vi "SVGen (FXP).vi"(7 "PWM  (Period)":fxp<+,32,10>, 8 "1/Vdc":fxp<+/-,16,10> format="%.16g", 9 "Vr3":fxp<+/-,32,12>, 10 "Vr2":fxp<+/-,32,12>, 11 "Vr1":fxp<+/-,32,12>) -> (0 "Tc":fxp<+/-,37,17> format="%.26g", 1 "PWM3":fxp<+,16,16>, 2 "PWM2":fxp<+,16,16>, 3 "PWM1":fxp<+,16,16>, 4 "Tb":fxp<+/-,37,17> format="%.26g", 5 "number":u8, 6 "Ta":fxp<+/-,37,17> format="%.26g")   [LabVIEW 2025]
uses:
  <vilib>/rvi/FXPMathLib/FxpMul/XNode/nifxpmath_Multiplier.xnode
  <vilib>/rvi/FXPMathLib/sim/FxpSim.dll
  <vilib>/Platform/TimedLoop/XDataNode/wakeup.ctl
  <vilib>/Platform/TimedLoop/XDataNode/XDNodeRunTimeDep.lvlib
  <vilib>/Platform/TimedLoop/XDataNode/nitl_modes.ctl
  <vilib>/Platform/TimedLoop/XDataNode/timing_clust.ctl
  <vilib>/platform/TimedLoop/XDataNode/XDataNode.xnode
  <vilib>/rvi/FXPMathLib/FxpAdd/XNode/nifxpmath_Add.xnode
panel:
  out "number":u8
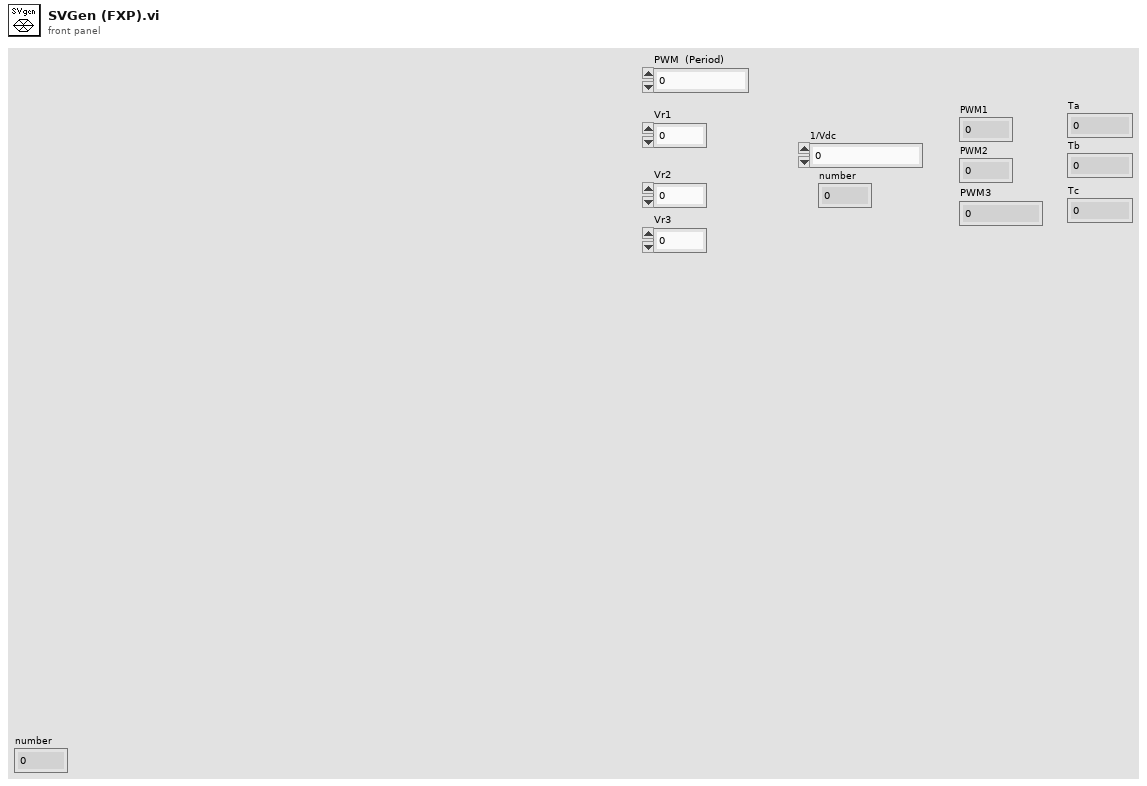
[diagram p1: front panel]
types:
  T1 = typedef "XDNodeRunTimeDep.lvlib/timing_clust.ctl" = cluster{"Expected End [f-1]":u64, "Actual End [f-1]":u64, "Finished Late? [f-1]":bool, "Expected End [i-1]":u64, "Actual End [i-1]":u64, "Finished Late? [i-1]":bool, "Expected Start [i]":u64, "Actual Start [i]":u64, "Expected Start [f]":u64, "Actual Start [f]":u64, "Source Name":string, "Structure Name":string, "Period":i64, "Deadline":i64, "Offset":i64, "Start":i64, "Priority":i32, "Timeout":i32, "Mode":T2, "Wakeup Reason":T3, "Error":errorcluster, "Source Type":string, "Secondary Source Type":string, "Global End Time":u64, "Global Start Time":u64, "Frame Duration":u64, "Iteration Duration":u64, "Assigned CPU":i32, "I/O Scan Engine Mode":u32}
  T2 = typedef "XDNodeRunTimeDep.lvlib/nitl_modes.ctl" = enum32{"No Change", "Process missed periods, maintain original phase", "Discard missed periods, maintain original phase", "Process missed periods, ignore original phase", "Discard missed periods, ignore original phase"}
  T3 = typedef "XDNodeRunTimeDep.lvlib/wakeup.ctl" = enum32{"Normal", "Aborted", "Asynchronous wakeup", "Timing source error", "Timed loop error", "Timeout"}
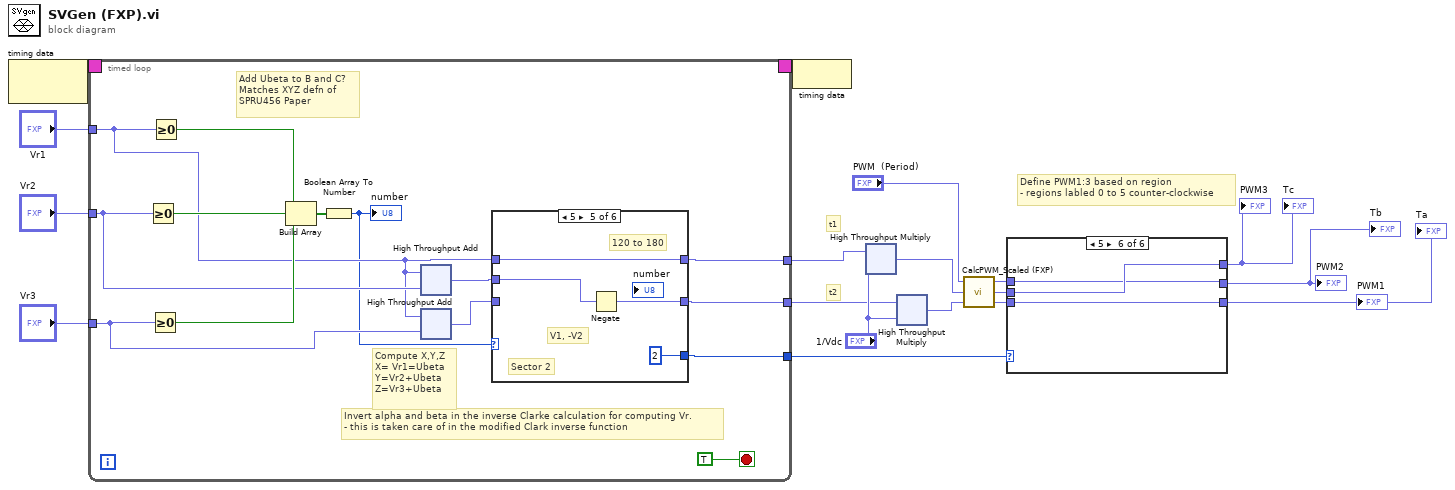
[diagram p0: block diagram]
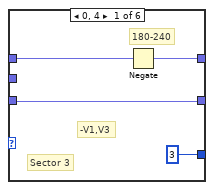
[diagram p2: hidden frame]
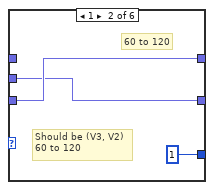
[diagram p3: hidden frame]
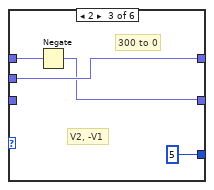
[diagram p4: hidden frame]
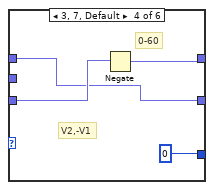
[diagram p5: hidden frame]
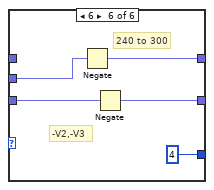
[diagram p6: hidden frame]
diagram:
  # "t2"
  # "t1"
  # "Define PWM1:3 based on region\n- regions labled 0 to 5 counter-clockwise"
  n1 = node-c288() -> (w18:T1)  [unwired: 1 out]
  n2 = timed-loop {
    timing: w18 -> [_]
    timing-out: [_] -> w17
    tunnel: [w20] -> w3
    tunnel: [w21] -> w7
    tunnel: [w22] -> w9
    tunnel: "Vr2" -> [w28]
    tunnel: "Vr1" -> [w25]
    tunnel: "Vr3" -> [w27]
    stop <- TRUE stop-if-true
    # "Compute X,Y,Z\nX= Vr1=Ubeta\nY=Vr2+Ubeta\nZ=Vr3+Ubeta"
    # "Add Ubeta to B and C?\nMatches XYZ defn of \nSPRU456 Paper"
    # "Invert alpha and beta in the inverse Clarke calculation for computing Vr.\n- this is taken care of in the modified Clark inverse function"
    n3 = Greater Or Equal To 0?(x=w28) -> (x >= 0?=w30:bool)
    n4 = Greater Or Equal To 0?(x=w27) -> (x >= 0?=w29:bool)
    n5 = Greater Or Equal To 0?(x=w25) -> (x >= 0?=w31:bool)
    n6 = Build Array(w31, w30, w29) -> (w32:bool[])
    n7 = Boolean Array To Number(Boolean array=w32) -> (number=w19:u8)
    "number" <- w19
    n8 = xnode "High Throughput Add"("x"=w25, "y"=w28) -> ("x+y"=w24:fxp<+/-,32,12>)
    n9 = xnode "High Throughput Add"("x"=w25, "y"=w27) -> ("x+y"=w23:fxp<+/-,32,12>)
    n10 = case shown="5" w19 {
      tunnel: [w36 w38 w41 w45 w50 w54] -> w22
      tunnel: w24 -> [_ w37 w41 _ w49 w55]
      tunnel: w23 -> [w33 w38 _ w46 _ w52]
      tunnel: [w33 w37 w40 w44 w48 w53] -> w21
      tunnel: w25 -> [w34 _ w42 w44 w50 _]
      tunnel: [3 1 5 0 2 4] -> w20
      frame 0, 4 {
        # "Sector 3"
        # "-V1,V3"
        # "180-240"
        n11 = Negate(x=w34) -> (-x=w36:fxp<+/-,33,13>)
      }
      frame 1 {
        # "Should be (V3, V2)\n60 to 120"
        # "60 to 120"
      }
      frame 2 {
        # "V2, -V1"
        # "300 to 0"
        n12 = Negate(x=w42) -> (-x=w40:fxp<+/-,33,13>)
      }
      frame 3, 7, Default {
        # "V2,-V1"
        # "0-60"
        n13 = Negate(x=w46) -> (-x=w45:fxp<+/-,33,13>)
      }
      frame 5 {
        # "Sector 2"
        # "V1, -V2"
        # "120 to 180"
        n14 = Negate(x=w49) -> (-x=w48:fxp<+/-,33,13>)
      }
      frame 6 {
        # "-V2,-V3"
        # "240 to 300"
        n15 = Negate(x=w55) -> (-x=w54:fxp<+/-,33,13>)
        n16 = Negate(x=w52) -> (-x=w53:fxp<+/-,33,13>)
      }
    }
  }
  n17 = node-c288(w17) -> ()
  n18 = xnode "High Throughput Multiply"("x"=w9, "y"="1/Vdc") -> ("x*y"=w10:fxp<+/-,32,12>)
  n19 = xnode "High Throughput Multiply"("x"=w7, "y"="1/Vdc") -> ("x*y"=w8:fxp<+/-,32,12>)
  n20 = call "CalcPWM_Scaled (FXP).vi"("T2"=w8, "T1"=w10, "PWM Period T"="PWM  (Period)") -> ("Ta"=w6:fxp<+/-,34,14>, "Tb"=w5:fxp<+/-,35,15>, "Tc"=w4:fxp<+/-,37,17>)
  n21 = case shown="5" w3 {
    tunnel: w6 -> [w61 w63 w67 w69 w71 w76]
    tunnel: [w61 w64 w66 w70 w72 w76] -> w2
    tunnel: [w60 w63 w67 w68 w73 w74] -> w16
    tunnel: w5 -> [w60 w64 w65 w68 w72 w75]
    tunnel: [w59 w62 w65 w69 w71 w75] -> w15
    tunnel: w4 -> [w59 w62 w66 w70 w73 w74]
    frame 0, Default {
    }
    frame 1 {
    }
    frame 2 {
    }
    frame 3 {
    }
    frame 4 {
    }
    frame 5 {
    }
  }
  "PWM3" <- w15
  "PWM1" <- w2
  "PWM2" <- w16
  "Tb" <- w16
  "Tc" <- w15
  "Ta" <- w2
